vi "APC_9049_ControlSettingsRaster.vi"(0 "SparkEnable":bool[](array[boolean]), 1 "InjectionEnable":bool[](array[boolean]), 2 "SparkTiming (DBTDC) loc":sgl, 3 "Speed (RPM)":sgl=1222.8582, 4 "9049 STATE":u8, 5 "PlsGen_Time_Config_In":T1) -> ()   [LabVIEW 2020]
doc: "This example demonstrates the procedure required to apply different NI-DAQmx Custom Scales to each virtual channel in a task. A DAQmx Task Property Node (Functions >> NI Measurements >> DAQmx - Data Acquisition >> DAQmx Advanced Task Options) is used to obtain the task's virtual channels. A DAQmx Channel Property Node (Functions >> NI Measurements >> DAQmx - Data Acquisition) is then used to set the custom scale for each virtual channel in the task.\n\nThe \"DAQmx Create Scale\" VI creates a custom scale for each channel in the channel list. *Note, make sure your Minimum and Maximum channel parameters are consistent with the range the scale will create."
panel:
  out "appended array":sgl[](array[numeric])
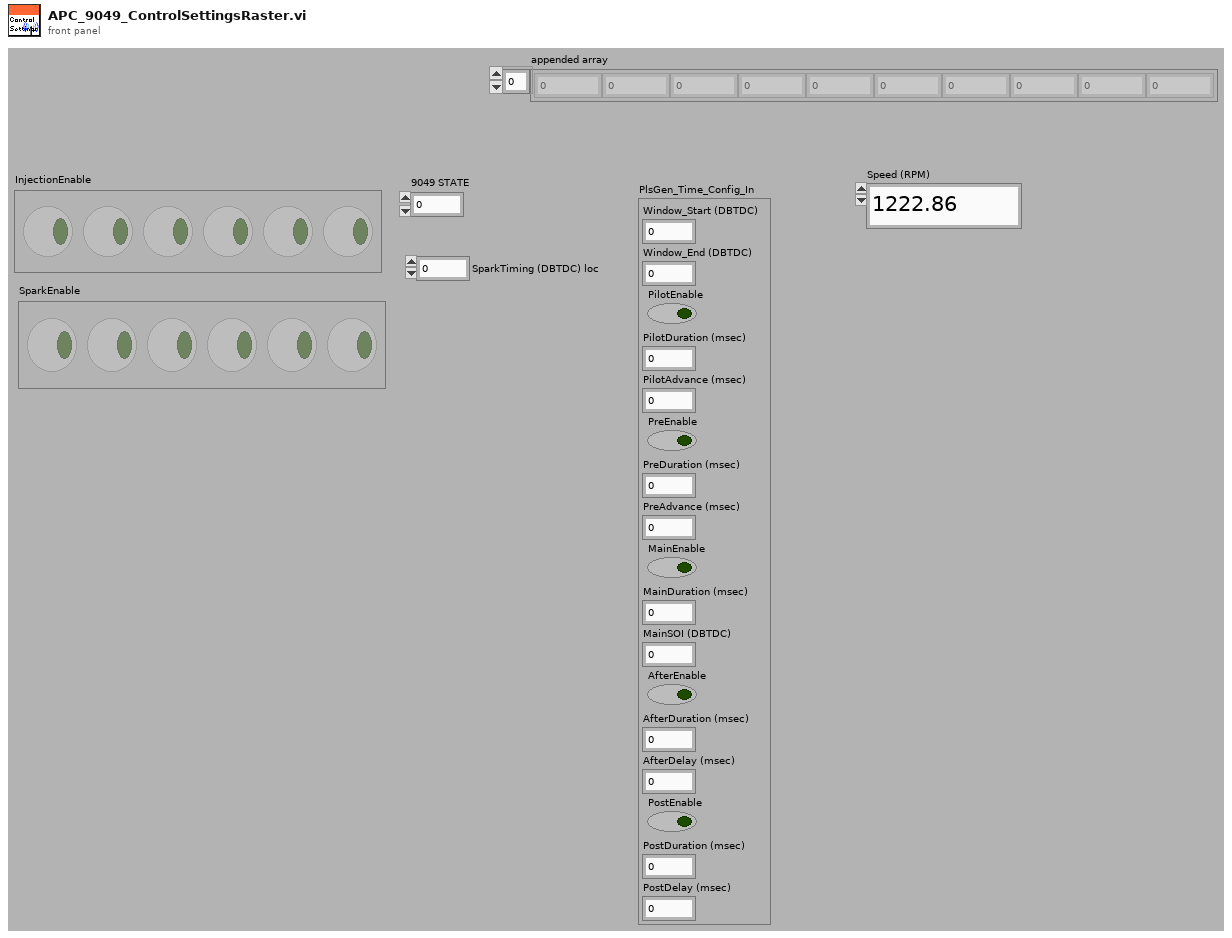
[diagram p1: front panel]
types:
  T1 = cluster{"Window_Start (DBTDC)":sgl, "Window_End (DBTDC)":sgl, "PilotEnable":bool, "PilotDuration (msec)":sgl, "PilotAdvance (msec)":sgl, "PreEnable":bool, "PreDuration (msec)":sgl, "PreAdvance (msec)":sgl, "MainEnable":bool, "MainDuration (msec)":sgl, "MainSOI (DBTDC)":sgl, "AfterEnable":bool, "AfterDuration (msec)":sgl, "AfterDelay (msec)":sgl, "PostEnable":bool, "PostDuration (msec)":sgl, "PostDelay (msec)":sgl}
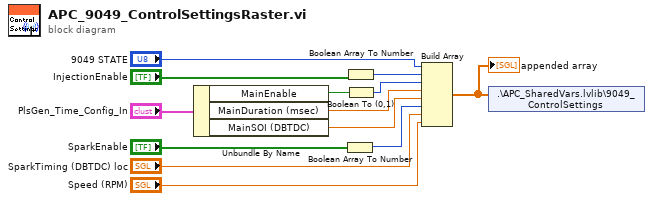
[diagram p0: block diagram]
diagram:
  n1 = Unbundle By Name("PlsGen_Time_Config_In") -> ("MainEnable"=w10:bool, "MainDuration (msec)"=w7:sgl, "MainSOI (DBTDC)"=w6:sgl)
  n2 = Boolean Array To Number(Boolean array="SparkEnable") -> (number=w5:u32)
  n3 = Boolean Array To Number(Boolean array="InjectionEnable") -> (number=w9:u32)
  n4 = Boolean To (0,1)(Boolean=w10) -> (0, 1=w8:i16)
  n5 = Build Array("9049 STATE", w9, w8, w7, w6, w5, "SparkTiming (DBTDC) loc", "Speed (RPM)") -> (w3:sgl[])
  "appended array" <- w3
  n6 = shared-variable ".\\APC_SharedVars.lvlib\\9049_ControlSettings"(w3) -> ()  [unwired: 1 in, 1 out]
